vi "Evaluate functional array.vi"(10 "Number Array":i32[](array[numeric]), 11 "Function Array":T1[](array[typedef])) -> (2 "Discard":bool, 3 "Complete Set":bool)   [LabVIEW 2023]
uses:
  ENUM_Type.ctl
panel:
  out "back counts":i32[](array[numeric])
  out "current counts":i32[](array[numeric])
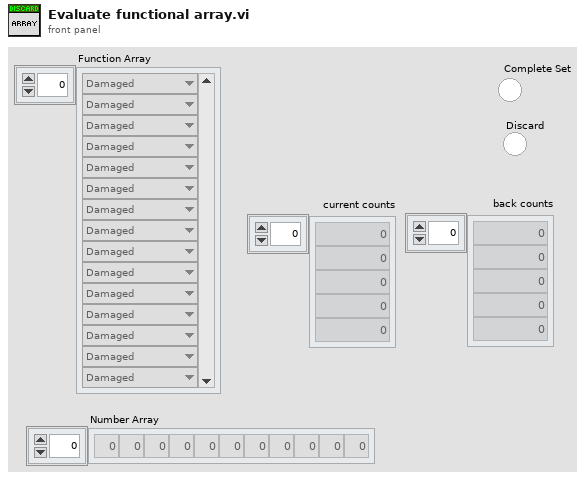
[diagram p1: front panel]
types:
  T1 = typedef "ENUM_Type.ctl" = enum16{"Damaged", "Operational", "Unknown"}
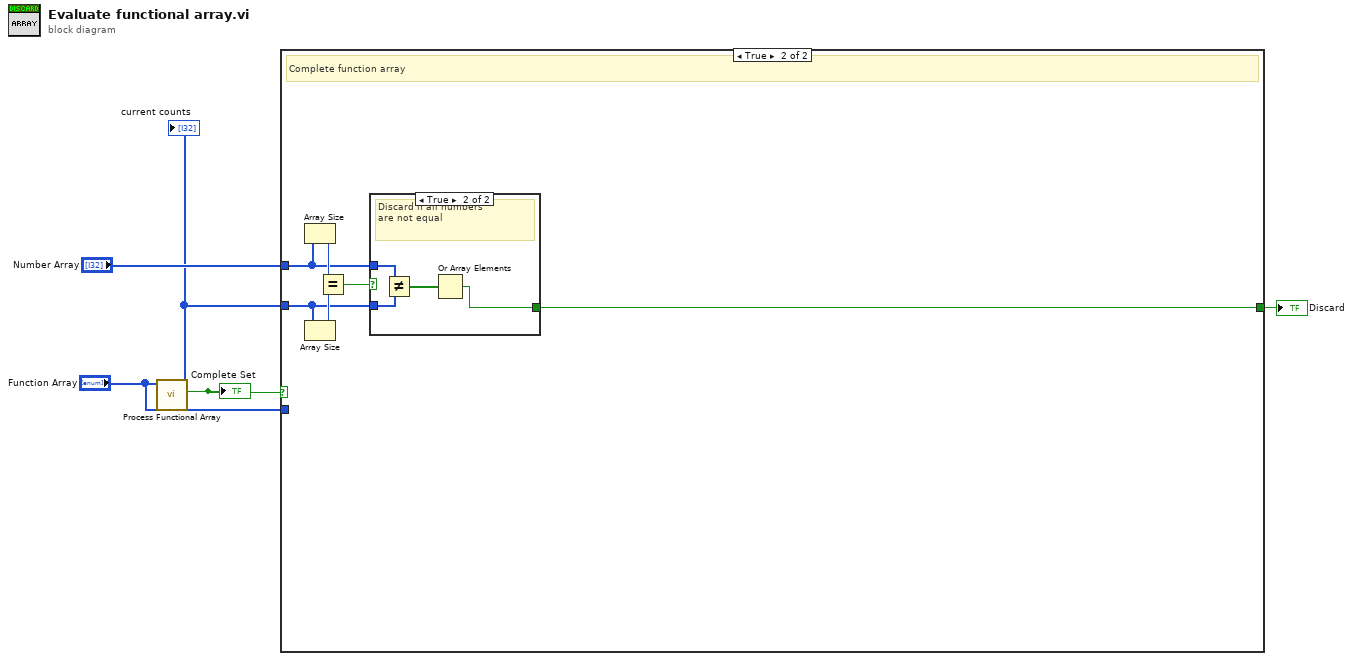
[diagram p0: block diagram]
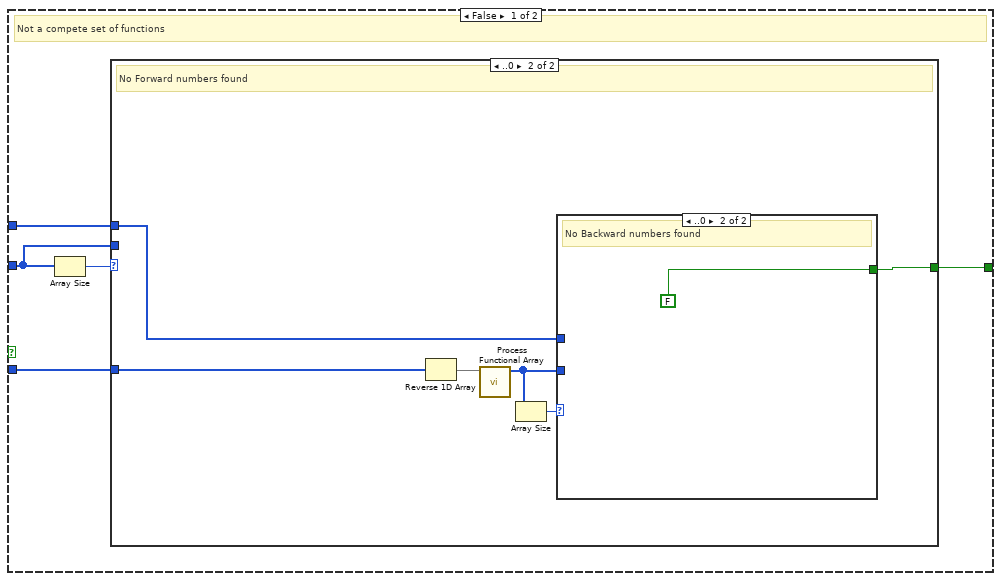
[diagram p2: hidden frame]
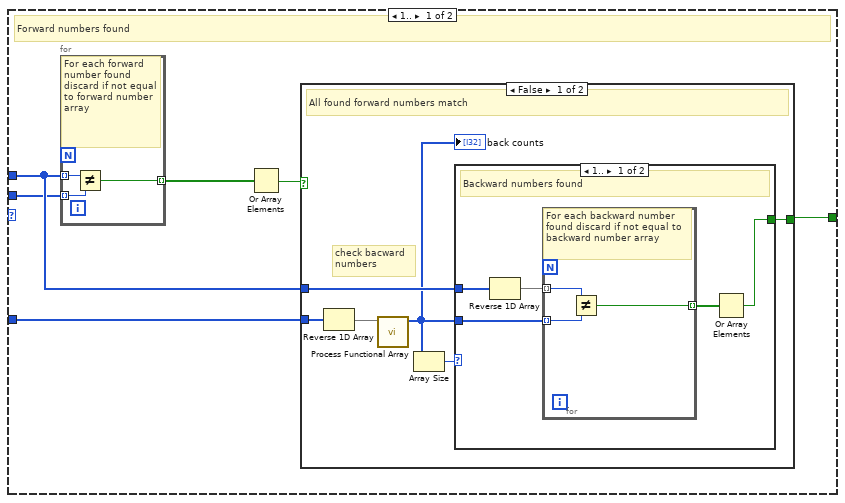
[diagram p3: hidden frame]
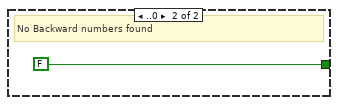
[diagram p4: hidden frame]
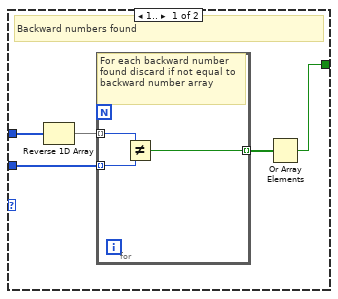
[diagram p6: hidden frame]
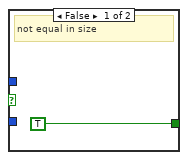
[diagram p7: hidden frame]
diagram:
  n1 = call "Process Functional Array.vi"("Function Array"="Function Array") -> ("Complete Array"=w2:bool, "Number Array"=w4:i32[])  [unwired: 9 in]
  "current counts" <- w4
  "Complete Set" <- w2
  n2 = case shown="True" w2 {
    tunnel: "Number Array" -> [w8 w51]
    tunnel: w4 -> [w7 w53]
    tunnel: [w9 w52] -> w3
    tunnel: "Function Array" -> [w6 _]
    frame False {
      # "Not a compete set of functions"
      n3 = Array Size(array=w7) -> (size(s)=w10:i32)
      n4 = case shown="..0" w10 {
        tunnel: w8 -> [w14 w41]
        tunnel: w7 -> [w12 _]
        tunnel: [w11 w39] -> w9
        tunnel: w6 -> [w13 w40]
        frame 1.. {
          # "Forward numbers found"
          n5 = for {
            tunnel: w12 -> [w19] mode=indexing
            tunnel: w14 -> [w18] mode=indexing
            tunnel: [w17] -> w16 mode=indexing
            # "For each forward number found discard if not equal to forward number array"
            n6 = Not Equal?(x=w18, y=w19) -> (x != y?=w17:bool)
          }
          n7 = Or Array Elements(Boolean array=w16) -> (logical OR=w15:bool)
          n8 = case shown="False" w15 {
            selector: w15 -> [_ w35]
            tunnel: w14 -> [w21 _]
            tunnel: w13 -> [w25 _]
            tunnel: [w22 w35] -> w11
            frame False {
              # "check bacward\nnumbers"
              # "All found forward numbers match"
              n9 = Reverse 1D Array(array=w25) -> (reversed array=w24:T1[])
              n10 = call "Process Functional Array.vi"("Function Array"=w24) -> ("Number Array"=w20:i32[])  [unwired: 9 in, 1 out]
              "back counts" <- w20
              n11 = Array Size(array=w20) -> (size(s)=w23:i32)
              n12 = case shown="1.." w23 {
                tunnel: [w26 FALSE] -> w22
                tunnel: w21 -> [w30 _]
                tunnel: w20 -> [w29 _]
                frame 1.. {
                  # "Backward numbers found"
                  n13 = Reverse 1D Array(array=w30) -> (reversed array=w28:i32[])
                  n14 = for {
                    tunnel: w29 -> [w32] mode=indexing
                    tunnel: w28 -> [w33] mode=indexing
                    tunnel: [w31] -> w27 mode=indexing
                    # "For each backward number found discard if not equal to backward number array"
                    n15 = Not Equal?(x=w33, y=w32) -> (x != y?=w31:bool)
                  }
                  n16 = Or Array Elements(Boolean array=w27) -> (logical OR=w26:bool)
                }
                frame ..0 {
                  # "No Backward numbers found"
                }
              }
            }
            frame True {
              # "Forward numbers do not match"
            }
          }
        }
        frame ..0 {
          # "No Forward numbers found"
          n17 = Reverse 1D Array(array=w40) -> (reversed array=w38:T1[])
          n18 = call "Process Functional Array.vi"("Function Array"=w38) -> ("Number Array"=w36:i32[])  [unwired: 9 in, 1 out]
          n19 = Array Size(array=w36) -> (size(s)=w37:i32)
          n20 = case shown="..0" w37 {
            tunnel: [w42 FALSE] -> w39
            tunnel: w41 -> [w46 _]
            tunnel: w36 -> [w45 _]
            frame 1.. {
              # "Backward numbers found"
              n21 = Reverse 1D Array(array=w46) -> (reversed array=w44:i32[])
              n22 = for {
                tunnel: w45 -> [w48] mode=indexing
                tunnel: w44 -> [w49] mode=indexing
                tunnel: [w47] -> w43 mode=indexing
                # "For each backward number found discard if not equal to backward number array"
                n23 = Not Equal?(x=w49, y=w48) -> (x != y?=w47:bool)
              }
              n24 = Or Array Elements(Boolean array=w43) -> (logical OR=w42:bool)
            }
            frame ..0 {
              # "No Backward numbers found"
            }
          }
        }
      }
    }
    frame True {
      # "Complete function array"
      n25 = Array Size(array=w51) -> (size(s)=w56:i32)
      n26 = Array Size(array=w53) -> (size(s)=w55:i32)
      n27 = Equal?(x=w56, y=w55) -> (x = y?=w54:bool)
      n28 = case shown="True" w54 {
        tunnel: w53 -> [_ w60]
        tunnel: [TRUE w58] -> w52
        tunnel: w51 -> [_ w61]
        frame False {
          # "not equal in size"
        }
        frame True {
          # "Discard if all numbers\nare not equal"
          n29 = Not Equal?(x=w61, y=w60) -> (x != y?=w59:bool[])
          n30 = Or Array Elements(Boolean array=w59) -> (logical OR=w58:bool)
        }
      }
    }
  }
  "Discard" <- w3
